vi "5900RW.vi"(1 "VISA resource name":refnum<visa-resource-name>="GPIB::1", 2 "ENTER STRING":string, 3 "Read ?":bool=TRUE, 4 "Write ?":bool=TRUE, 8 "# bytes\nto read":i32=200) -> (6 "Characters Read":string, 9 "error out":errorcluster)   [LabVIEW 2022 SP3]
doc: "A device connected to a GPIB bus can be written to or be read from using this VI. Select the GPIB address of the device, choose Read or Write or both, type in the characters to be written, and run the VI. If you choose both Read and Write, the VI will write to the device first, then read from the device. Before using this VI you should initialize the GPIB address according to the device's specifications with the \"GPIB Initialization\" function."
panel:
  out "return count":u32
  out "Write Status":string
  out "Read Status":string
  # "Select  the GPIB address of the device, choose Read or Write or both, type in the characters to be written, and run the VI. If you choose both Read and Write, the VI will write to the device first, then read from the device.  Before using this VI you should initialize the GPIB address according to the device's specifications with the \"GPIB Initialization\" function."
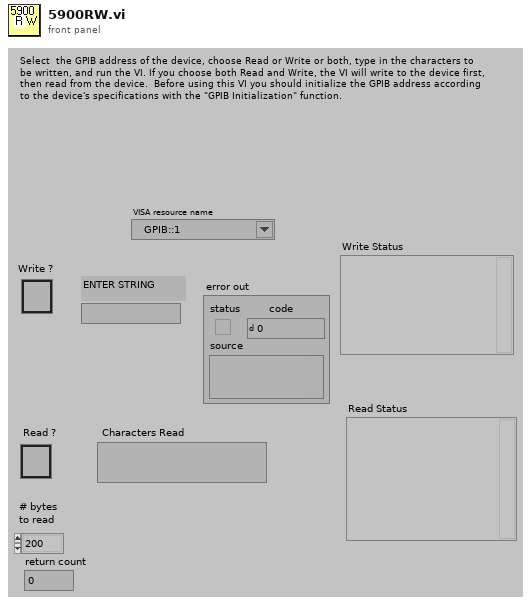
[diagram p1: front panel]
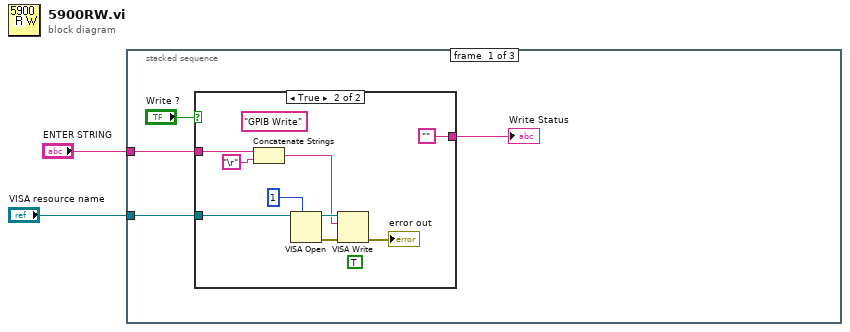
[diagram p0: block diagram]
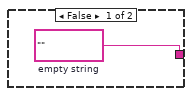
[diagram p2: hidden frame]
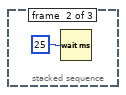
[diagram p3: hidden frame]
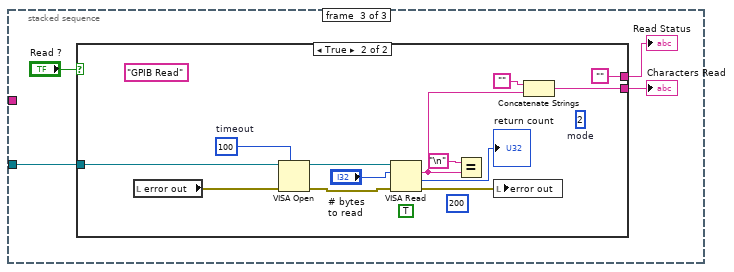
[diagram p4: hidden frame]
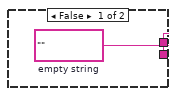
[diagram p5: hidden frame]
diagram:
  n1 = stacked-sequence {
    tunnel: "ENTER STRING" -> [w4 _ _]
    tunnel: "VISA resource name" -> [w3 _ w18]
    frame #0 {
      n2 = case shown="True" "Write ?" {
        tunnel: [w7 ""] -> w5
        tunnel: w4 -> [_ w15]
        tunnel: w3 -> [_ w14]
        frame False {
          w7 = ""  # empty string
        }
        frame True {
          (unwired) TRUE
          (unwired) "GPIB Write"
          n3 = Concatenate Strings(w15, "\r") -> (w10:string)
          n4 = VISA Open(timeout (0)=1, VISA resource name=w14) -> (VISA resource name=w13:refnum<visa-resource-name>, error out=w12:errorcluster)  [unwired: 1 in, 2 out]
          n5 = VISA Write(VISA resource name=w13, write buffer=w10, error in (no error)=w12) -> (error out=→"error out":errorcluster)  [unwired: 2 out]
        }
      }
      "Write Status" <- w5
    }
    frame #1 {
      n6 = Wait (ms)(milliseconds to wait=25) -> ()  [unwired: 1 out]
    }
    frame #2 {
      n7 = case shown="True" "Read ?" {
        tunnel: [w22 w32] -> w19
        tunnel: [w22 ""] -> w20
        tunnel: w18 -> [_ w31]
        frame False {
          w22 = ""  # empty string
        }
        frame True {
          (unwired) u32 200 ("General Settings:Timeout Value")
          (unwired) TRUE
          (unwired) "GPIB Read"
          w33 = u32 100  # timeout
          (unwired) 2  # mode
          n8 = local read "error out"() -> (w30:errorcluster)
          n9 = VISA Open(timeout (0)=w33, error in (no error)=w30, VISA resource name=w31) -> (VISA resource name=w27:refnum<visa-resource-name>, error out=w26:errorcluster)  [unwired: 2 out]
          n10 = VISA Read(VISA resource name=w27, byte count="# bytes\nto read", error in (no error)=w26) -> (read buffer=w24:string, return count=→"return count":u32, error out=w29:errorcluster)  [unwired: 1 out]
          n11 = Equal?(x="\n", y=w24) -> ()  [unwired: 1 out]
          n12 = local write "error out"(w29) -> ()
          n13 = Concatenate Strings("", w24) -> (w32:string)
        }
      }
      "Read Status" <- w20
      "Characters Read" <- w19
    }
  }
